vi "RyanTestComp.vi"(10 "NEW":dbl[](array[numeric]), 11 "OLD":dbl[](array[numeric])) -> (3 "Boolean":bool)   [LabVIEW 2016]
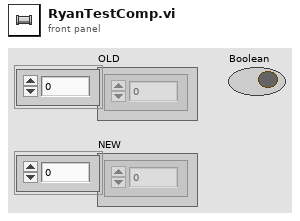
[diagram p1: front panel]
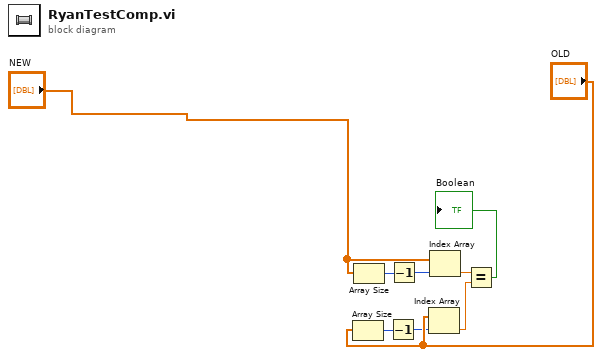
[diagram p0: block diagram]
diagram:
  n1 = Array Size(array="OLD") -> (size(s)=w5:i32)
  n2 = Array Size(array="NEW") -> (size(s)=w1:i32)
  n3 = Decrement(x=w5) -> (x-1=w6:i32)
  n4 = Decrement(x=w1) -> (x-1=w2:i32)
  n5 = Index Array(array="OLD", index=w6) -> (element=w8:dbl)
  n6 = Index Array(array="NEW", index=w2) -> (element=w4:dbl)
  n7 = Equal?(x=w4, y=w8) -> (x = y?=→"Boolean":bool)
